vi "Get MSG.vi"(11 "Queue in":T1) -> (0 "error out":errorcluster, 2 "more than five":bool, 3 "MSG for servo":T2={"Command"=enum."Initialize", "Data"=variant(dbl[] [])})   [LabVIEW 2017, in "Servo drive module.lvlib"]
doc: "Extracts a message from master controler.\nparams:\nQueue reference\nreturns: \nCommand cluster for a servo drive."
uses:
  Servo drive module.lvlib
  ctl/Servo MSG.ctl
  ctl/Servo commands.ctl
  Messenger service/Data types/Mailbox address.ctl
  Messenger service/MessengerLib.lvlib
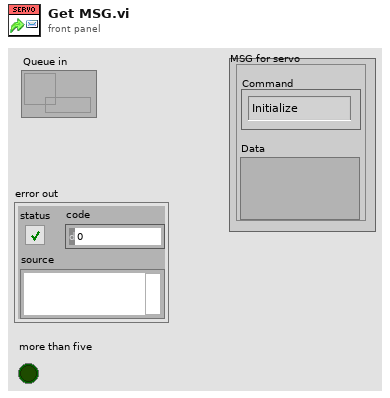
[diagram p1: front panel]
types:
  T1 = typedef "MessengerLib.lvlib/Mailbox address.ctl" = refnum<queue>
  T2 = typedef "Servo drive module.lvlib/Servo MSG.ctl" = cluster{"Command":T3, "Data":variant}
  T3 = typedef "Servo drive module.lvlib/Servo commands.ctl" = enum16{"Initialize", "Update", "Move by", "Move to", "Stop", "Ignore", "End"}
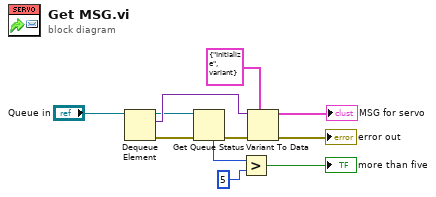
[diagram p0: block diagram]
diagram:
  n1 = Dequeue Element(queue="Queue in") -> (queue out=w2:T1, element=w4:variant, error out=w1:errorcluster)  [unwired: 2 in, 1 out]
  n2 = Get Queue Status(queue=w2, error in (no error)=w1) -> (error out=w8:errorcluster, # elements in queue=w7:i32)  [unwired: 1 in, 6 out]
  n3 = Greater?(x=w7, y=5) -> (0:→"more than five":bool)
  n4 = Variant To Data(error in=w8, type=T2 {"Command"=enum."Initialize", "Data"=variant(dbl[] [])} ("MSG to Servo"), Variant=w4) -> (data=→"MSG for servo":T2, error out=→"error out":errorcluster)
